vi "CollectVideoPacket.vi"(8 "error in (no error)":errorcluster, 11 "CameraTestingProxyAPI in":refnum<class "CameraTestingProxyAPI.lvclass">) -> (0 "error out":errorcluster, 2 "VideoDataPacket":T1, 3 "CameraTestingProxyAPI out":refnum<class "CameraTestingProxyAPI.lvclass">)   [LabVIEW 2020, in "CameraTestingProxy.lvlib" / "CameraTestingProxyAPI.lvclass"]
uses:
  CameraTestingProxyAPI.lvclass
  ICameraTestingProxy/ICameraTestingProxy/TypeDef/VideoDataPacket.ctl
  ICameraTestingProxy/ICameraTestingProxy/TypeDef/VideoFrameData.ctl
  CameraTestingProxyAPI.lvclass/CameraTestingProxyAPI.ctl
  ICameraTestingProxy/ICameraTestingProxy/ICameraTestingProxy.lvclass
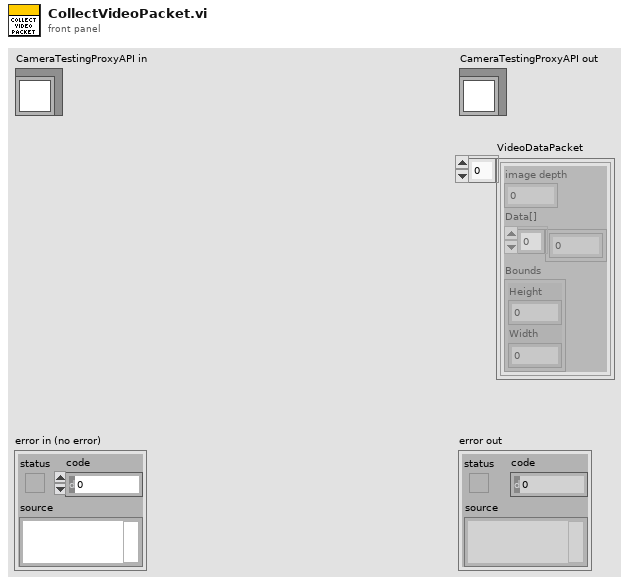
[diagram p1: front panel]
types:
  T1 = typedef "ICameraTestingProxy.lvlib/ICameraTestingProxy.lvclass/VideoDataPacket.ctl" = T2[]
  T2 = typedef "ICameraTestingProxy.lvlib/ICameraTestingProxy.lvclass/VideoFrameData.ctl" = cluster{"image depth":i32, "Data[]":u8[], "Bounds":cluster{"Height":i16, "Width":i16}}
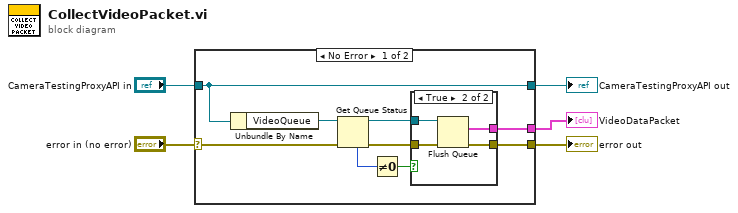
[diagram p0: block diagram]
diagram:
  n1 = case shown="No Error" "error in (no error)" {
    selector: "error in (no error)" -> [w14 w21]
    tunnel: [w6 w21] -> w1
    tunnel: [w13 w20] -> w4
    tunnel: "CameraTestingProxyAPI in" -> [w13 w20]
    tunnel: [w7 _] -> w2
    frame No Error {
      n2 = Unbundle By Name(w13) -> ("VideoQueue"=w12:refnum<queue>)
      n3 = Get Queue Status(queue=w12, error in (no error)=w14) -> (queue out=w9:refnum<queue>, error out=w8:errorcluster, # elements in queue=w11:i32)  [unwired: 1 in, 5 out]
      n4 = Not Equal To 0?(x=w11) -> (x != 0?=w10:bool)
      n5 = case shown="True" w10 {
        tunnel: w9 -> [_ w19]
        tunnel: w8 -> [w15 w18]
        tunnel: [_ w17] -> w7
        tunnel: [w15 w16] -> w6
        frame False {
        }
        frame True {
          n6 = Flush Queue(queue=w19, error in (no error)=w18) -> (remaining elements=w17:T2[], error out=w16:errorcluster)  [unwired: 1 out]
        }
      }
    }
    frame Error {
    }
  }
  "error out" <- w1
  "CameraTestingProxyAPI out" <- w4
  "VideoDataPacket" <- w2
